vi "GE ALGO.vi"() -> ()   [LabVIEW 2016]
panel:
  out "a":cdb[][](array[numeric])
  out "Array 2":dbl[][](array[numeric])
  out "arccos(x) 2":dbl[](array[numeric])
  out "decimated array 7":cdb[](array[numeric])
  out "decimated array 6":cdb[](array[numeric])
  out "decimated array 5":cdb[](array[numeric])
  out "subarray 2":cdb[](array[numeric])
  out "r * e^(i*theta)":cdb[](array[numeric])
  out "Array 3":cdb[](array[numeric])
  out "Array":dbl[](array[numeric])
  out "x*y":dbl
  out "Samples for normal":dbl[](array[numeric])
  out "NON REC Magnitude 2":dbl[](array[numeric])
  out "NON REC":dbl[](array[numeric])
  out "Waveform Graph":dbl[](graph)
  out "Magnitude":dbl[](array[numeric])
  out "Angle":dbl[](array[numeric])
  in  "Phase":dbl
  in  "Number Of samples":i32
  in  "Frequency":dbl
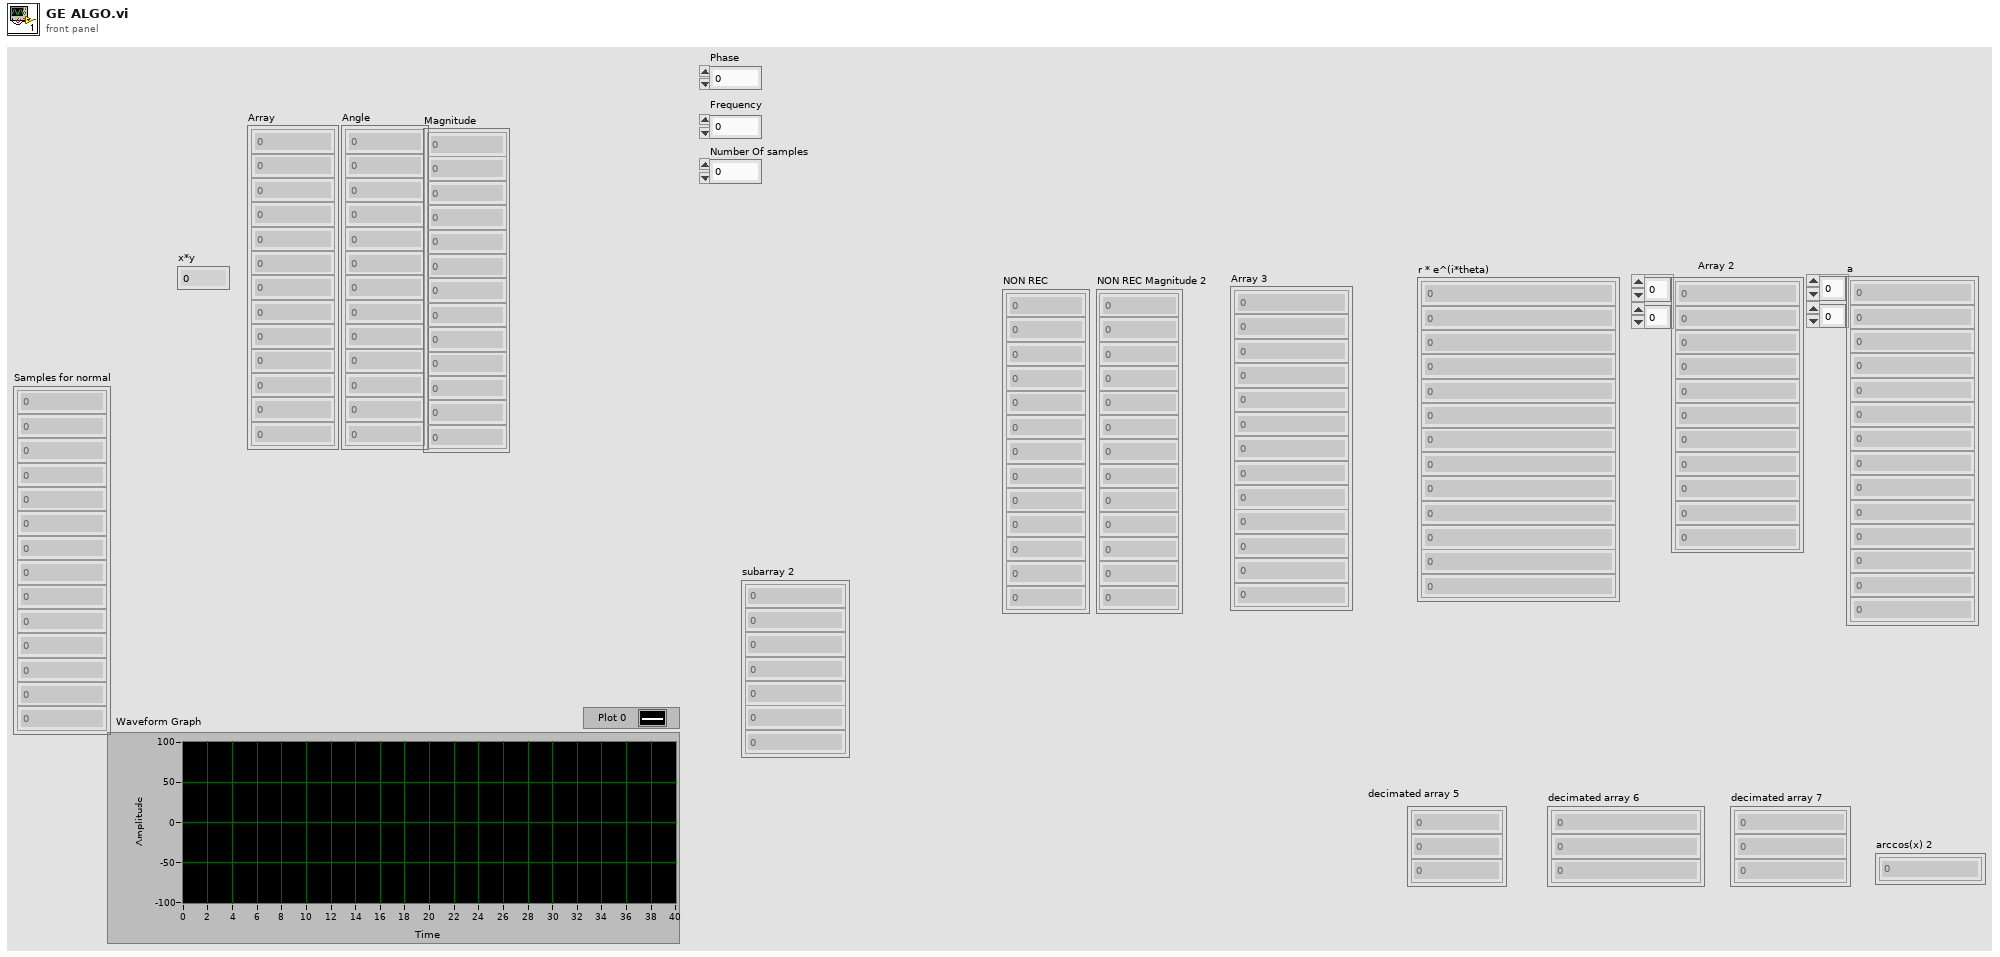
[diagram p1: front panel]
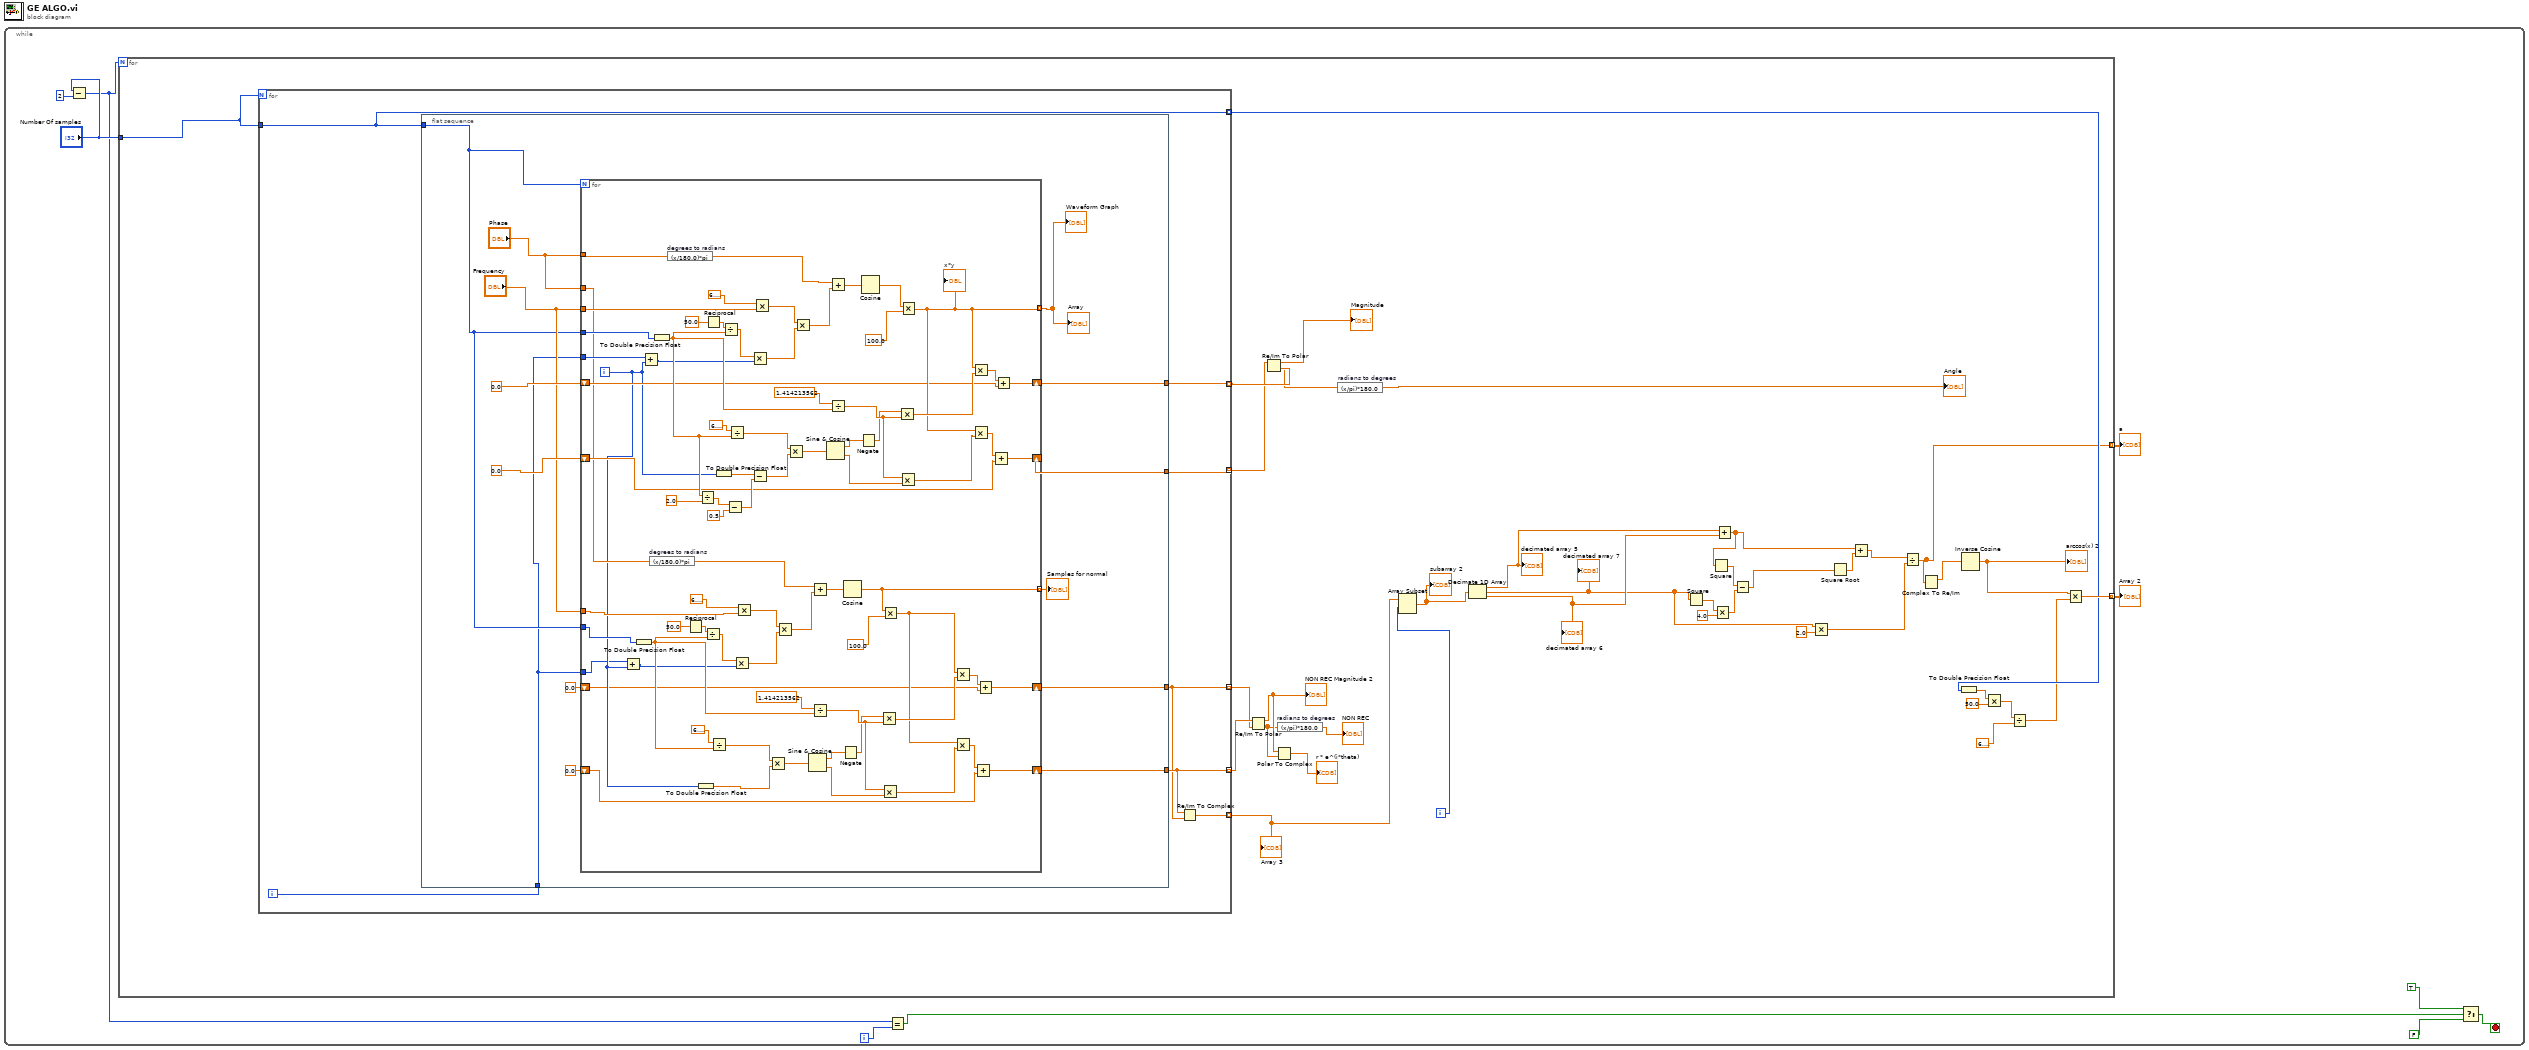
[diagram p0: block diagram]
diagram:
  n1 = while {
    i -> [w6]
    stop <- w8 stop-if-true
    n2 = Subtract(x="Number Of samples", y=2) -> (x-y=w3:i32)
    n3 = for {
      N: w3 -> [_]
      tunnel: "Number Of samples" -> [w21]
      tunnel: [w18] -> w2 mode=indexing
      tunnel: [w11] -> w1 mode=indexing
      i -> [w19]
      n4 = for {
        N: w21 -> [_]
        tunnel: w21 -> [w49]
        tunnel: [w54] -> w48 mode=indexing
        tunnel: [w53] -> w47 mode=indexing
        tunnel: [w51] -> w41 mode=indexing
        tunnel: [w52] -> w43 mode=indexing
        tunnel: [w50] -> w20 mode=indexing
        tunnel: [w49] -> w13 mode=indexing
        i -> [w55]
        n5 = flat-sequence {
          tunnel: w49 -> [w62]
          tunnel: w55 -> [w61]
          tunnel: [w65] -> w54
          tunnel: [w66] -> w53
          tunnel: [w58] -> w51
          tunnel: [w57] -> w52
          frame #0 {
            n6 = for {
              N: w62 -> [_]
              tunnel: "Frequency" -> [w135]
              tunnel: [w119] -> w67 mode=indexing
              tunnel: w62 -> [w137]
              tunnel: "Phase" -> [w111]
              shift-right: [w117] -> w66
              shift-left: 0.0 -> [w114]
              shift-right: [w118] -> w65
              shift-left: 0.0 -> [w116]
              tunnel: w61 -> [w107]
              tunnel: "Phase" -> [w82]
              tunnel: "Frequency" -> [w81]
              tunnel: w62 -> [w80]
              tunnel: w61 -> [w78]
              shift-right: [w77] -> w58
              shift-left: 0.0 -> [w74]
              shift-right: [w76] -> w57
              shift-left: 0.0 -> [w75]
              tunnel: [w70] -> w56 mode=indexing
              i -> [w79]
              n7 = Add(x=w78, y=w79) -> (x+y=w83:i32)
              n8 = To Double Precision Float(number=w80) -> (double precision float=w92:dbl)
              n9 = Add(x=w107, y=w79) -> (x+y=w108:i32)
              n10 = expression code="(x/180.0)*pi" "degrees to radians"(w82) -> (w86:dbl)
              n11 = To Double Precision Float(number=w137) -> (double precision float=w122:dbl)
              n12 = expression code="(x/180.0)*pi" "degrees to radians"(w111) -> (w112:dbl)
              n13 = Reciprocal(x=50.0) -> (1/x=w99:dbl)
              n14 = To Double Precision Float(number=w79) -> (double precision float=w73:dbl)
              n15 = Divide(x=w122, y=2.0) -> (x/y=w125:dbl)
              n16 = Divide(x=w99, y=w92) -> (x/y=w102:dbl)
              n17 = Reciprocal(x=50.0) -> (1/x=w136:dbl)
              n18 = Divide(x=6.283185307179586, y=w92) -> (x/y=w97:dbl)
              n19 = To Double Precision Float(number=w79) -> (double precision float=w127:dbl)
              n20 = Divide(x=w136, y=w122) -> (x/y=w141:dbl)
              n21 = Subtract(x=w125, y=0.5) -> (x-y=w123:dbl)
              n22 = Divide(x=6.283185307179586, y=w122) -> (x/y=w133:dbl)
              n23 = Multiply(x=w102, y=w83) -> (x*y=w105:dbl)
              n24 = Multiply(x=6.283185307179586, y=w81) -> (x*y=w106:dbl)
              n25 = Multiply(x=w141, y=w108) -> (x*y=w144:dbl)
              n26 = Subtract(x=w127, y=w123) -> (x-y=w132:dbl)
              n27 = Multiply(x=6.283185307179586, y=w135) -> (x*y=w145:dbl)
              n28 = Multiply(x=w97, y=w73) -> (x*y=w96:dbl)
              n29 = Multiply(x=w106, y=w105) -> (x*y=w104:dbl)
              n30 = Multiply(x=w133, y=w132) -> (x*y=w131:dbl)
              n31 = Multiply(x=w145, y=w144) -> (x*y=w143:dbl)
              n32 = Sine & Cosine(0:w96) -> (1:w85:dbl, 2:w93:dbl)
              n33 = Add(x=w86, y=w104) -> (x+y=w101:dbl)
              n34 = Divide(x=1.414213562, y=w92) -> (x/y=w94:dbl)
              n35 = Sine & Cosine(0:w131) -> (1:w110:dbl, 2:w128:dbl)
              n36 = Add(x=w112, y=w143) -> (x+y=w140:dbl)
              n37 = Divide(x=1.414213562, y=w122) -> (x/y=w129:dbl)
              n38 = Negate(x=w85) -> (-x=w84:dbl)
              n39 = Cosine(x=w101) -> (cos(x)=w70:dbl)
              n40 = Negate(x=w110) -> (-x=w109:dbl)
              n41 = Cosine(x=w140) -> (cos(x)=w138:dbl)
              n42 = Multiply(x=w84, y=w94) -> (x*y=w90:dbl)
              n43 = Multiply(x=w94, y=w93) -> (x*y=w91:dbl)
              n44 = Multiply(x=w70, y=100.0) -> (x*y=w89:dbl)
              n45 = Multiply(x=w109, y=w129) -> (x*y=w120:dbl)
              n46 = Multiply(x=w129, y=w128) -> (x*y=w121:dbl)
              n47 = Multiply(x=w138, y=100.0) -> (x*y=w119:dbl)
              "x*y" <- w119
              n48 = Multiply(x=w89, y=w90) -> (x*y=w88:dbl)
              n49 = Multiply(x=w89, y=w91) -> (x*y=w87:dbl)
              n50 = Multiply(x=w119, y=w120) -> (x*y=w115:dbl)
              n51 = Multiply(x=w119, y=w121) -> (x*y=w113:dbl)
              n52 = Add(x=w87, y=w75) -> (x+y=w76:dbl)
              n53 = Add(x=w88, y=w74) -> (x+y=w77:dbl)
              n54 = Add(x=w113, y=w114) -> (x+y=w117:dbl)
              n55 = Add(x=w115, y=w116) -> (x+y=w118:dbl)
            }
            "Waveform Graph" <- w67
            "Samples for normal" <- w56
            "Array" <- w67
          }
        }
        n56 = Re/Im To Complex(1:w51, 2:w52) -> (0:w50:cdb)
      }
      "Array 3" <- w20
      n57 = Re/Im To Polar(2:w41, 3:w43) -> (0:w39:dbl[], 1:w40:dbl[])
      "NON REC Magnitude 2" <- w40
      n58 = Re/Im To Polar(2:w48, 3:w47) -> (0:w45:dbl[], 1:→"Magnitude":dbl[])
      n59 = Polar To Complex(1:w39, 2:w40) -> (0:→"r * e^(i*theta)":cdb[])
      n60 = expression code="(x/pi)*180.0" "radians to degrees"(w39) -> (→"NON REC":dbl[])
      n61 = expression code="(x/pi)*180.0" "radians to degrees"(w45) -> (→"Angle":dbl[])
      n62 = Array Subset(array=w20, index=w19) -> (w25:cdb[])  [unwired: 1 in]
      "subarray 2" <- w25
      n63 = Decimate 1D Array(w25) -> (w24:cdb[], w22:cdb[], w23:cdb[])
      "decimated array 5" <- w24
      "decimated array 6" <- w23
      "decimated array 7" <- w22
      n64 = Square(x=w22) -> (x^2=w34:cdb[])
      n65 = Multiply(x=w34, y=4.0) -> (x*y=w33:cdb[])
      n66 = Add(x=w24, y=w23) -> (x+y=w36:cdb[])
      n67 = Square(x=w36) -> (x^2=w32:cdb[])
      n68 = Subtract(x=w32, y=w33) -> (x-y=w31:cdb[])
      n69 = Multiply(x=w22, y=2.0) -> (x*y=w28:cdb[])
      n70 = Square Root(x=w31) -> (sqrt(x)=w37:cdb[])
      n71 = Add(x=w36, y=w37) -> (x+y=w30:cdb[])
      n72 = Divide(x=w30, y=w28) -> (x/y=w11:cdb[])
      n73 = Complex To Re/Im(x + iy=w11) -> (x=w27:dbl[])  [unwired: 1 out]
      n74 = To Double Precision Float(number=w13) -> (double precision float=w14:dbl[])
      n75 = Inverse Cosine(1:w27) -> (0:w26:dbl[])
      "arccos(x) 2" <- w26
      n76 = Multiply(x=w14, y=50.0) -> (x*y=w15:dbl[])
      n77 = Divide(x=w15, y=6.283185307179586) -> (x/y=w12:dbl[])
      n78 = Multiply(x=w26, y=w12) -> (x*y=w18:dbl[])
    }
    "Array 2" <- w2
    "a" <- w1
    n79 = Equal?(x=w3, y=w6) -> (x = y?=w7:bool)
    n80 = Select(t=TRUE, s=w7, f=FALSE) -> (s? t:f=w8:bool)
  }
